vi "Eurotherm - Read Auto Tune Status.vi"(0 "Eurotherm Setup In":T2={"Communication"={"Com Port"=1, "Address"=1, "Baud Rate"=9600}, "Name"="", "Enable"=FALSE, "Max Set Point"=0.0, "Min Set Point"=0.0, "Units"="", "Graph Data"=0, "Sensor type"=enum."RhFe", "Calibration File Path"=path "", "Conversion Type"=enum."Linear"} {"Min Set Point" format="%.3f"; "Max Set Point" format="%.3f"; "Communication"."Baud Rate" items=["300"=300, "600"=600, "1200"=1200, "2400"=2400, "4800"=4800, "9600 (default)"=9600, "19200"=19200, "38400"=38400, "57600"=57600, "76800"=76800, "115200"=115200, "230400"=230400]; "Communication"."Com Port" min=1 max=255; "Communication"."Address" min=1 max=99}, 11 "error in (no error)":errorcluster) -> (4 "Eurotherm Setup Out":T2={"Communication"={"Com Port"=1, "Address"=1, "Baud Rate"=9600}, "Name"="", "Enable"=FALSE, "Max Set Point"=0.0, "Min Set Point"=0.0, "Units"="", "Graph Data"=0, "Sensor type"=enum."RhFe", "Calibration File Path"=path "", "Conversion Type"=enum."Linear"} {"Min Set Point" format="%.3f"; "Max Set Point" format="%.3f"; "Communication"."Baud Rate" items=["300"=300, "600"=600, "1200"=1200, "2400"=2400, "4800"=4800, "9600 (default)"=9600, "19200"=19200, "38400"=38400, "57600"=57600, "76800"=76800, "115200"=115200, "230400"=230400]; "Communication"."Com Port" min=1 max=255; "Communication"."Address" min=1 max=99}, 8 "Auto Tune State":bool, 15 "error out":errorcluster)   [LabVIEW 2011]
uses:
  Eurotherm - Controls/Eurotherm - Setup.ctl
  Eurotherm - Controls/Eurotherm - Communication.ctl
  Common/Utilities/Controls - Com Ports/Com Port - Numeric.ctl
  Eurotherm - Controls/Eurotherm - Address.ctl
  Common/Utilities/Controls - Com Ports/Com Port - Baud Rate.ctl
  Common/Utilities - System/Sensors/Sensors - Controls/Sensors - Temperature Sensor Type.ctl
  Common/Utilities - System/Sensors/Sensors - Controls/Sensors - Conversion Type.ctl
  Eurotherm - Controls/Eurotherm - AutoTune State.ctl
panel:
  out "Auto Tune State":T1
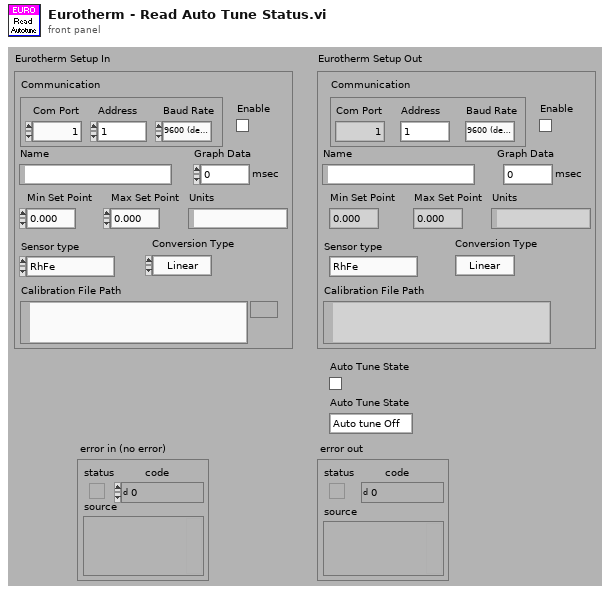
[diagram p1: front panel]
types:
  T1 = typedef "Eurotherm - AutoTune State.ctl" = enum16{"Auto tune Off", "Auto Tune On"}
  T2 = typedef "Eurotherm - Setup.ctl" = cluster{"Communication":T3, "Name":string, "Enable":bool, "Max Set Point":dbl, "Min Set Point":dbl, "Units":string, "Graph Data":u32, "Sensor type":T7, "Calibration File Path":path, "Conversion Type":T8}
  T3 = typedef "Eurotherm - Communication.ctl" = cluster{"Com Port":T4, "Address":T5, "Baud Rate":T6}
  T4 = typedef "Com Port - Numeric.ctl" = i32
  T5 = typedef "Eurotherm - Address.ctl" = u8
  T6 = typedef "Com Port - Baud Rate.ctl" = u32
  T7 = typedef "Sensors - Temperature Sensor Type.ctl" = enum16{"RhFe", "Pt", "K type thermocouple", "W5 type thermocouple", "No Conversion"}
  T8 = typedef "Sensors - Conversion Type.ctl" = enum16{"Linear", "Spline"}
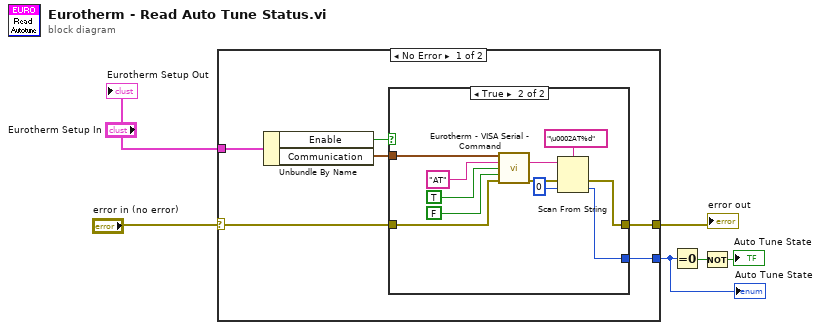
[diagram p0: block diagram]
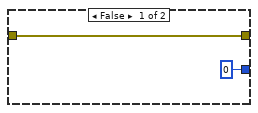
[diagram p2: hidden frame]
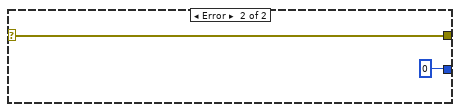
[diagram p3: hidden frame]
diagram:
  n1 = case shown="No Error" "error in (no error)" {
    selector: "error in (no error)" -> [w12 w27]
    tunnel: [w11 w27] -> w5
    tunnel: [w7 u8 0 ("default value 1")] -> w1
    tunnel: "Eurotherm Setup In" -> [w8 _]
    frame No Error {
      n2 = Unbundle By Name(w8) -> ("Enable"=w9:bool, "Communication"=w10:T3)
      n3 = case shown="True" w9 {
        tunnel: w12 -> [w14 w25]
        tunnel: [w14 w18] -> w11
        tunnel: w10 -> [_ w21]
        tunnel: [u8 0 w15] -> w7
        frame False {
        }
        frame True {
          n4 = call "Eurotherm - VISA Serial - Command.vi"("VISA resource name In (String)"=w21, "Command"="AT", "Read Reply"=TRUE, "Close Session"=FALSE, "error in (no error)"=w25) -> ("Reply"=w17:string, "error out"=w19:errorcluster)  [unwired: 8 in, 1 out]
          n5 = Scan From String(format string="\u0002AT%d", input string=w17, error in=w19, default 1=u8 0) -> (error out=w18:errorcluster, output 1=w15:u8)  [unwired: 1 in, 2 out]
        }
      }
    }
    frame Error {
    }
  }
  "error out" <- w5
  "Auto Tune State" <- w1
  n6 = Equal To 0?(x=w1) -> (x = 0?=w3:bool)
  n7 = Not(x=w3) -> (.not. x?=→"Auto Tune State":bool)
  "Eurotherm Setup Out" <- "Eurotherm Setup In"
